vi "MKS_UNIT (SubVI).vi"(8 "error in (no error)":errorcluster, 10 "MKS UNITS":string(combo)="MBAR" caption="Units", 11 "Cluster in":T1 caption="Cluster 2" {"parity (0:none)" items=["None", "Odd", "Even", "Mark", "Space"]; "BAUDE RATE" items=["38400"=38400, "19200"=19200, "9600"=9600, "4800"=4800]}) -> (0 "error out":errorcluster, 3 "result string":string)   [LabVIEW 2020]
uses:
  INITIALIZATION.ctl
  <vilib>/Instr/_visa.llb/VISA Configure Serial Port (Instr).vi
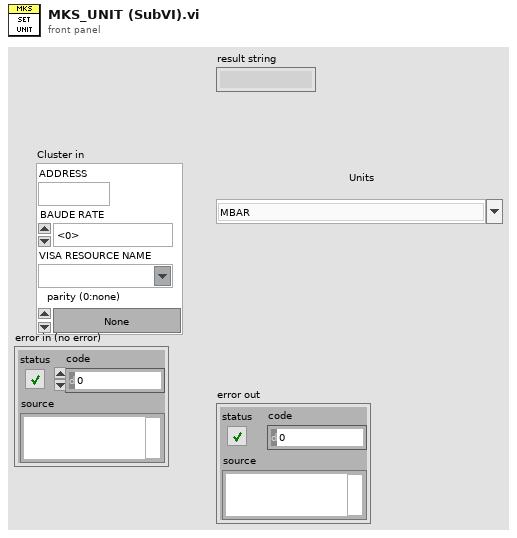
[diagram p1: front panel]
types:
  T1 = typedef "INITIALIZATION.ctl" = cluster{"ADDRESS":string, "BAUDE RATE":u32, "VISA RESOURCE NAME":refnum<visa-resource-name>, "parity (0:none)":u16}
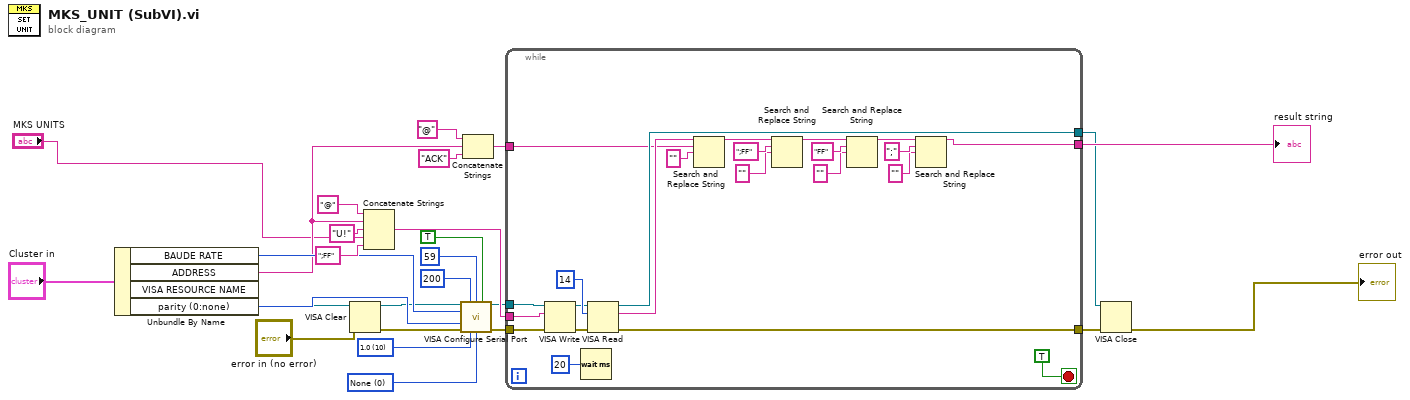
[diagram p0: block diagram]
diagram:
  w14 = u16 0 items=["None", "XON/XOFF", "RTS/CTS", "XON/XOFF & RTS/CTS", "DTR/DSR", "XON/XOFF & DTR/DSR"] ("flow control (0:none)")
  w20 = u16 10 items=["1.0"=10, "1.5"=15, "2.0"=20] ("stop bits (10: 1 bit)")
  n1 = Unbundle By Name("Cluster in") -> ("BAUDE RATE"=w19:u32, "ADDRESS"=w12:string, "VISA RESOURCE NAME"=w4:refnum<visa-resource-name>, "parity (0:none)"=w13:u16)
  n2 = VISA Clear(VISA resource name=w4, error in (no error)="error in (no error)") -> (VISA resource name out=w5:refnum<visa-resource-name>, error out=w3:errorcluster)
  n3 = Concatenate Strings("@" ("string"), w12, "U!" ("string"), "MKS UNITS", ";FF" ("string")) -> (w27:string)
  n4 = call-poly "VISA Configure Serial Port"("VISA resource name"=w5, "timeout (10sec)"=u32 200, "termination char\n(0xA = '\\n' = LF)"=u8 59, "Enable Termination\nChar (T)"=TRUE ("Enable Termination\nChar (T)"), "baud rate (9600)"=w19, "parity (0:none)"=w13, "error in (no error)"=w3, "stop bits (10: 1 bit)"=w20, "flow control (0:none)"=w14) -> ("VISA resource name out"=w16:refnum<visa-resource-name>, "error out"=w15:errorcluster)  [unwired: 5 in]
  n5 = Concatenate Strings("@" ("search string"), w12, "ACK" ("string")) -> (w6:string)
  n6 = while {
    tunnel: w15 -> [w50]
    tunnel: [w48] -> w11
    tunnel: w16 -> [w49]
    tunnel: [w47] -> w24
    tunnel: w27 -> [w38]
    tunnel: w6 -> [w37]
    tunnel: [w28] -> w25
    stop <- TRUE stop-if-true
    n7 = VISA Write(VISA resource name=w49, write buffer=w38, error in (no error)=w50) -> (VISA resource name out=w30:refnum<visa-resource-name>, error out=w29:errorcluster)  [unwired: 1 out]
    n8 = Wait (ms)(milliseconds to wait=u32 20) -> ()  [unwired: 1 out]
    n9 = VISA Read(VISA resource name=w30, byte count=u32 14, error in (no error)=w29) -> (VISA resource name out=w47:refnum<visa-resource-name>, read buffer=w44:string, error out=w48:errorcluster)  [unwired: 1 out]
    n10 = Search and Replace String(input string=w44, search string=w37, replace string="" ("replace string (\"\")")) -> (result string=w42:string)  [unwired: 5 in, 3 out]
    n11 = Search and Replace String(input string=w42, search string=";FF", replace string="" ("replace string (\"\")")) -> (result string=w33:string)  [unwired: 5 in, 3 out]
    n12 = Search and Replace String(input string=w33, search string="FF", replace string="" ("replace string (\"\")")) -> (result string=w32:string)  [unwired: 5 in, 3 out]
    n13 = Search and Replace String(input string=w32, search string=";", replace string="" ("replace string (\"\")")) -> (result string=w28:string)  [unwired: 5 in, 3 out]
  }
  "result string" <- w25
  n14 = VISA Close(VISA resource name=w24, error in (no error)=w11) -> (error out=→"error out":errorcluster)
